vi "SQL_在指定表中查找ALL数据.vi"(8 "error in (no error)":errorcluster caption="错误输入（无错误）", 10 "表名":string="d7", 11 "字段（产品编码）":string="d7") -> (0 "error out":errorcluster caption="错误输出", 3 "SQL_在指定表中指定字段插入数据":string)   [LabVIEW 2014]
doc: "该模板用于创建子VI。"
uses:
  <vilib>/addons/database/NI_Database_API.lvlib
  <vilib>/addons/database/Connection.llb/DB Tools Open Connec (String).vi
  <vilib>/addons/database/Connection.llb/Conn Execute.vi
  <vilib>/addons/database/Recordset.llb/Rec Destroy - Connection.vi
panel:
  out "error out 2":errorcluster
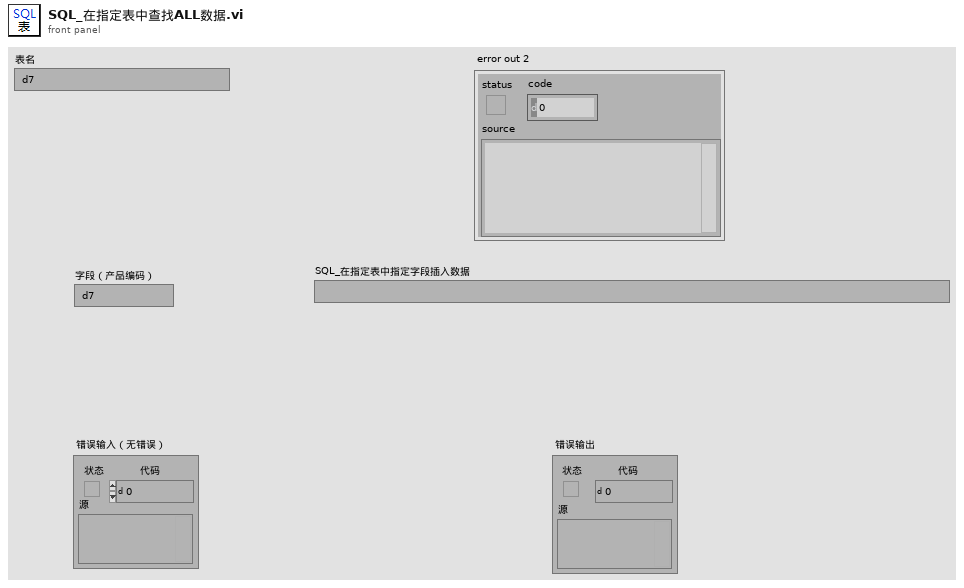
[diagram p1: front panel]
types:
  T1 = typedef "NI_Database_API.lvlib/Conn ObjectReference.ctl" = refnum<k1>
  T2 = typedef "NI_Database_API.lvlib/Rec ObjectReference.ctl" = refnum<k1>
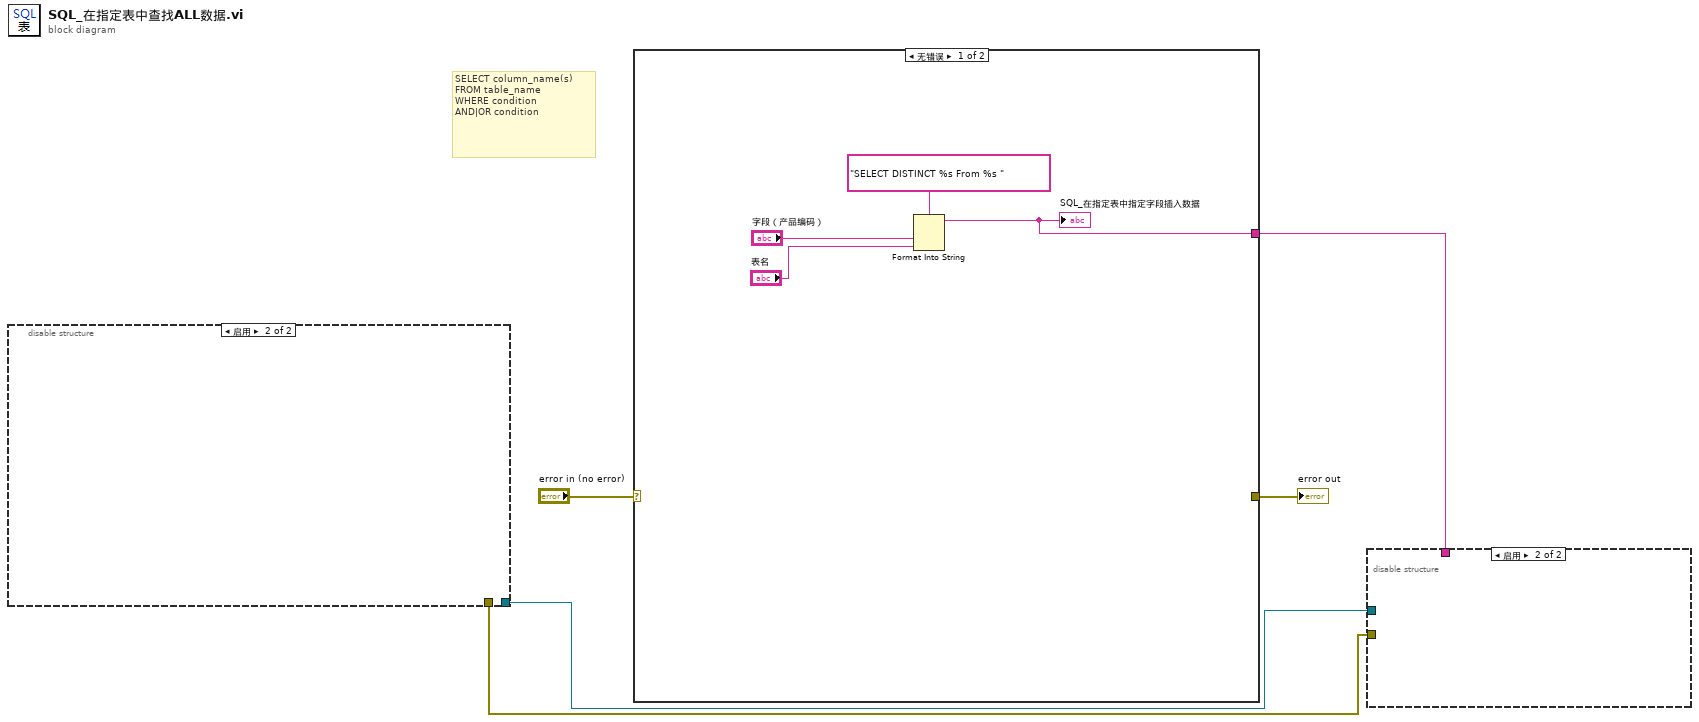
[diagram p0: block diagram]
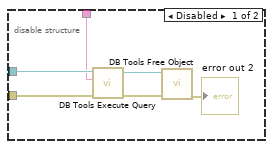
[diagram p2: hidden frame]
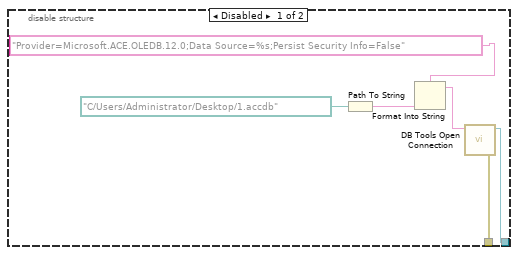
[diagram p3: hidden frame]
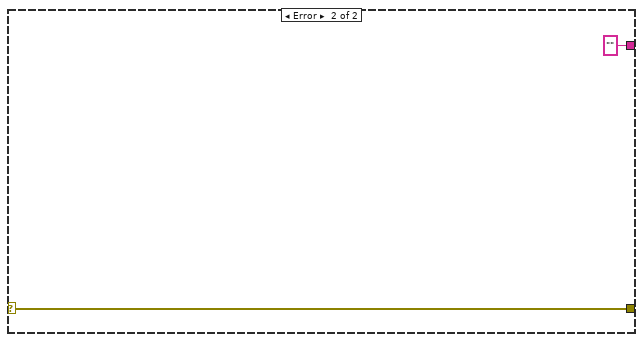
[diagram p4: hidden frame]
diagram:
  # "SELECT column_name(s)\nFROM table_name\nWHERE condition\nAND|OR condition"
  n1 = disable-structure shown="启用" {
    disable-tunnel: [w8 _] -> w3
    disable-tunnel: [w6 _] -> w2
    frame Disabled {
      n2 = Path To String(path=path "C:/Users/Administrator/Desktop/1.accdb" ("路径")) -> (string=w11:string)
      n3 = Format Into String(format string="Provider=Microsoft.ACE.OLEDB.12.0;Data Source=%s;Persist Security Info=False" ("初始字符串"), w11) -> (resulting string=w10:string)  [unwired: 2 in, 1 out]
      n4 = call-poly <vilib>:"DB Tools Open Connection.vi"("connection information"=w10) -> ("error out"=w6:errorcluster, "connection reference"=w8:T1)  [unwired: 7 in]
    }
    frame Enabled {
    }
  }
  n5 = case shown="无错误" "error in (no error)" {
    selector: "error in (no error)" -> [_ w17]
    tunnel: [_ w17] -> w4
    tunnel: [w13 ""] -> w1
    frame No Error {
      n6 = Format Into String(format string="SELECT DISTINCT %s From %s ", "字段（产品编码）", "表名") -> (resulting string=w13:string)  [unwired: 2 in, 1 out]
      "SQL_在指定表中指定字段插入数据" <- w13
    }
    frame Error {
    }
  }
  "error out" <- w4
  n7 = disable-structure shown="启用" {
    disable-tunnel: w3 -> [w20 _]
    disable-tunnel: w2 -> [w19 _]
    disable-tunnel: w1 -> [w18 _]
    frame Disabled {
      n8 = call-poly <vilib>:"DB Tools Execute Query.vi"("error in (no error)"=w19, "SQL query"=w18, "connection reference"=w20) -> ("error out"=w22:errorcluster, "recordset reference"=w23:T2)  [unwired: 5 in]
      n9 = call-poly <vilib>:"DB Tools Free Object.vi"("error in (no error)"=w22, "recordset reference"=w23) -> ("error out"=→"error out 2":errorcluster)  [unwired: 8 in, 1 out]
    }
    frame Enabled {
    }
  }
